vi "Read seq_state.vi"(8 "error in (no error)":errorcluster, 11 "gController in":refnum<class "gController.lvclass">) -> (0 "error out":errorcluster, 2 "seq_state":refnum<queue>, 3 "gController out":refnum<class "gController.lvclass">)   [LabVIEW 2017, in "Controller.lvlib" / "gController.lvclass"]
uses:
  gController.lvclass
  Sequencer/sequenceState.ctl
  Controller.lvlib
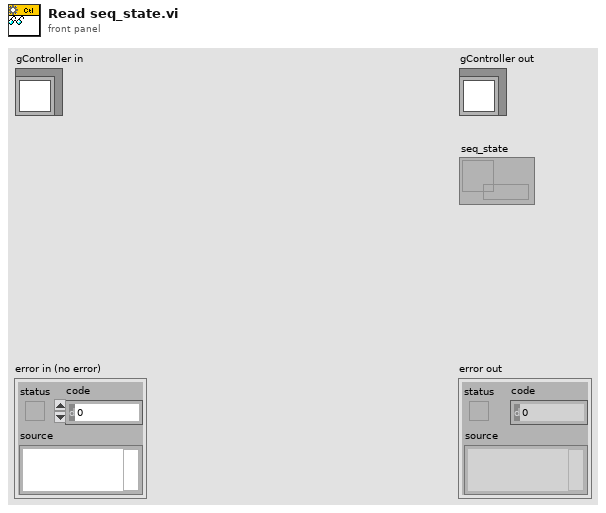
[diagram p1: front panel]
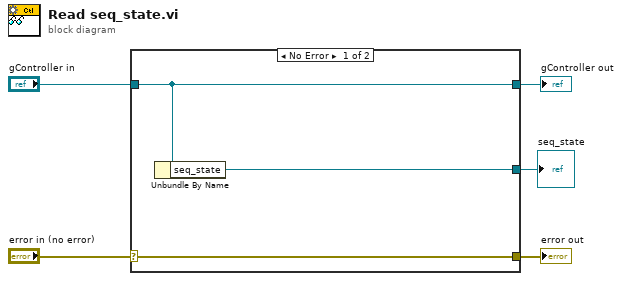
[diagram p0: block diagram]
diagram:
  n1 = case shown="No Error" "error in (no error)" {
    selector: "error in (no error)" -> [w8 w9]
    tunnel: [w8 w9] -> w4
    tunnel: [w7 w10] -> w2
    tunnel: "gController in" -> [w7 w10]
    tunnel: [w6 _] -> w1
    frame No Error {
      n2 = Unbundle By Name(w7) -> ("seq_state"=w6:refnum<queue>)
    }
    frame Error {
    }
  }
  "error out" <- w4
  "gController out" <- w2
  "seq_state" <- w1
